vi "app - Ross Thing.vi"() -> ()   [LabVIEW 2012]
uses:
  <vilib>/event_ctls.llb/eventvkey.ctl
  freq file -- file select control.ctl
  freq file -- file select folder control.ctl
  cursor winow.ctl
  fit function selector control.ctl
  countdown control.ctl
  cursor window action.ctl
  container action.ctl
  cursor action.ctl
  save-read action.ctl
  file -- 9w path.vi
  file -- open-create folder.vi
panel:
  in  "main folder":path=path "\\\\rus-one\\newdata/data/Ultrasound/Experiment/ProbeTest/Birdcage/YBCO_6_opt"
  out "Plot: argan":T1(graph)
  in  "Tab : other":enum32{"indicators", "other"}(tab)=enum."other"
  in  "file 2 (red)":T2={"from file "="2011_mo", "load"=TRUE, "read from file list"=3, "folder kind"=enum."monitor"} {"read from file list" items=["795_mo", "1348_mo", "1644_mo", "2011_mo", "2100_mo"]}
  in  "file 1 (blue)":T2={"from file "="2011_mo", "load"=TRUE, "read from file list"=4, "folder kind"=enum."monitor"} {"read from file list" items=["586_mo", "792_mo", "1644_mo", "1865_mo", "2011_mo", "2730_mo"]}
  out "time (min)":dbl=808.9068825910931
  in  "open (o)":bool
  in  "plot (p)":bool
  in  "plot type":T4(ring)=enum."plot vs Temperature"
  out "temperature (K)":dbl=39.718
  out "Magnetic Field (T)":dbl=0.65596
  in  "sweep folder 2":u16(ring)=18 items=["1_test", "2_heating_0T", "3_field_to_5T", "4_cooling_5T", "5_heating_5T", "6_cooling_10T", "7_heating_10T", "8_cooling_1T", "9_heating_2T", "10_test", "11_heating_0T", "12_heating_0T", "14_field_to_5T", "15_field_to_0T", "16_field_to_10T", "17_field_to_0T", "18_field_to_10T", "19_cooling_10T", "20_heating_10T"]
  in  "sweep folder 1":u16(ring)=17 items=["1_test", "2_heating_0T", "3_field_to_5T", "4_cooling_5T", "5_heating_5T", "6_cooling_10T", "7_heating_10T", "8_cooling_1T", "9_heating_2T", "10_test", "11_heating_0T", "12_heating_0T", "14_field_to_5T", "15_field_to_0T", "16_field_to_10T", "17_field_to_0T", "18_field_to_10T", "19_cooling_10T", "20_heating_10T"]
  out "folder --OK":bool=TRUE
  out "file 2 -- OK":bool=TRUE
  out "file 1 -- OK":bool=TRUE
  out "best fit parameters":dbl[](array[numeric])=[2010.73341095214, -73.95493561675569, 194.69833504908257]
  in  "fit dataset":enum16{"fit blue dataset", "fit red  dataset"}(ring)
  in  "fit using":T5=enum."einstein"
  out "current index":dbl=2087.4915004944774
  out "Char":i16=51
  out "VKey":T6
  in  "Tab: timer":enum32{"timer ON", "timer OFF"}(tab)
  in  "timer  \"update\"":dbl(slide)=31059.326000000176 min=-209828747.99999982 max=2129711151.0 step=0.010000000000000002 scale=0.0..300.0 scale format="%#3_3f"
  in  "Tab : all":enum32{"everything", "everything else"}(tab)
  out "Plot: temp vs time":cluster{dbl[], dbl[]}[](graph)
  out "Plot: gamma":cluster{dbl[], dbl[]}[](graph)=[{array[2829 elements], array[2829 elements]}, {[15.988, 15.895, 15.895, 15.863, 15.823, 15.791, 15.753, 15.714, 15.682, 15.645, 15.614, 15.576, 15.545, 15.508, 15.472, 15.441, 15.405, 15.375, 15.339, 15.309, 15.274, 15.245, 15.209, 15.175, 15.146, 15.112, 15.084, 15.05, 15.022, 14.988, 14.96, 14.926, 14.892, 14.864, 14.83, 14.802, 14.769, 14.741, 14.708, 14.675, 14.648, 14.616, 14.589, 14.557, 14.53, 14.499, 14.472, 14.441, 14.41, 14.384, 14.353, 14.327, 14.297, 14.272, 14.242, 14.212, 14.188, 14.158, 14.134, 14.108, 14.091, 14.082, 14.085, 14.104, 14.141, 14.186, 14.259, 14.332, 14.435, 14.532, 14.66, 14.776, 14.923, 15.078, 15.212, 15.375, 15.514, 15.68, 15.818, 15.983, 16.144, 16.275, 16.429, 16.554, 16.697, 16.814, 16.947, 17.054, 17.177, 17.295, 17.39, 17.498, 17.585, 17.685, 17.767, 17.86, 17.951, 18.024, 18.111, 18.181, 18.265, 18.333, 18.415, 18.496, 18.562, 18.643, 18.711, 18.792, 18.861, 18.945, 19.016, 19.102, 19.188, 19.262, 19.352, 19.428, 19.52, 19.598, 19.694, 19.773, 19.87, 19.968, 20.051, 20.151, 20.234, 20.335, 20.419, 20.521, 20.622, 20.706, 20.807, 20.891, 20.992, 21.075, 21.175, 21.258, 21.355, 21.453, 21.534, 21.63, 21.709, 21.804, 21.882, 21.975, 22.068, 22.144, 22.235, 22.31, 22.399, 22.473, 22.562, 22.635, 22.722, 22.81, 22.882, 22.969, 23.041, 23.127, 23.199, 23.285, 23.372, 23.458, 23.545, 23.631, 23.631, 23.717, 23.791, 23.849, 23.922, 23.995, 24.083, 24.157, 24.231, 24.32, 24.394, 24.47, 24.56, 24.635, 24.71, 24.817, 24.924, 25.016, 25.123, 25.216, 25.324, 25.417, 25.526, 25.619, 25.728, 25.821, 25.931, 26.025, 26.134, 26.229, 26.339, 26.448, 26.543, 26.652, 26.746, 26.856, 26.95, 27.06, 27.154, 27.264, 27.359, 27.468, 27.563, 27.673, 27.782, 27.877, 27.987, 28.082, 28.193, 28.288, 28.399, 28.493, 28.605, 28.701, 28.812, 28.909, 29.021, 29.118, 29.231, 29.344, 29.442, 29.556, 29.654, 29.768, 29.868, 29.984, 30.082, 30.2, 30.299, 30.417, 30.518, 30.636, 30.738, 30.857, 30.976, 31.08, 31.2, 31.304, 31.425, 31.529, 31.652, 31.757, 31.881, 31.987, 32.111, 32.217, 32.342, 32.45, 32.576, 32.702, 32.811, 32.938, 33.047, 33.176, 33.286, 33.415, 33.526, 33.656, 33.768, 33.9, 34.012, 34.144, 34.276, 34.391, 34.525, 34.639, 34.773, 34.889], [0.02015, 0.02965, 0.02923, 0.02683, 0.02605, 0.02852, 0.02316, 0.0243, 0.02505, 0.02987, 0.02439, 0.02523, 0.02405, 0.02435, 0.02757, 0.02568, 0.02492, 0.02492, 0.02742, 0.02961, 0.03389, 0.02022, 0.02642, 0.03056, 0.02673, 0.03264, 0.0206, 0.02411, 0.02374, 0.02762, 0.02435, 0.02784, 0.02951, 0.0205, 0.02387, 0.02656, 0.02196, 0.02912, 0.02801, 0.02441, 0.0273, 0.02807, 0.02433, 0.02863, 0.02677, 0.02849, 0.02892, 0.02528, 0.02579, 0.02902, 0.02854, 0.02679, 0.02086, 0.02834, 0.02825, 0.03102, 0.02966, 0.02864, 0.02638, 0.02732, 0.02698, 0.02975, 0.0277, 0.02987, 0.02672, 0.02935, 0.02685, 0.02704, 0.03128, 0.02306, 0.02001, 0.0269, 0.02455, 0.03277, 0.02896, 0.03053, 0.02583, 0.02668, 0.02805, 0.02642, 0.02325, 0.03759, 0.03048, 0.03819, 0.02667, 0.02874, 0.0294, 0.02773, 0.02917, 0.02492, 0.02754, 0.02348, 0.02597, 0.01897, 0.02318, 0.03016, 0.00123, 0.02855, 0.02386, 0.02476, 0.02543, 0.02862, 0.02883, 0.02667, 0.02727, 0.02846, 0.02979, 0.02773, 0.02675, 0.0282, 0.02506, 0.02126, 0.02901, 0.0228, 0.02825, 0.02834, 0.02612, 0.02559, 0.02108, 0.02742, 0.02585, 0.03164, 0.02195, 0.02756, 0.02835, 0.02988, 0.0272, 0.02663, 0.01825, 0.02181, 0.02802, 0.02825, 0.02726, 0.02242, 0.02544, 0.02547, 0.02545, 0.02683, 0.02214, 0.02583, 0.02758, 0.02628, 0.03141, 0.03234, 0.02479, 0.03261, 0.02449, 0.03183, 0.02764, 0.02827, 0.02715, 0.02372, 0.02469, 0.02966, 0.02697, 0.02742, 0.03078, 0.02539, 0.02565, 0.03029, 0.0221, 0.02024, 0.02769, 0.02882, 0.02943, 0.02649, 0.02713, 0.02892, 0.0248, 0.02651, 0.02454, 0.02248, 0.02563, 0.02862, 0.02788, 0.03423, 0.02351, 0.02644, 0.02672, 0.02602, 0.03194, 0.02539, 0.02141, 0.02587, 0.03321, 0.02646, 0.02893, 0.0267, 0.02558, 0.02828, 0.03125, 0.02901, 0.027, 0.02611, 0.03, 0.02445, 0.02946, 0.03169, 0.03087, 0.0278, 0.03122, 0.02918, 0.03277, 0.02628, 0.03193, 0.02932, 0.02643, 0.0297, 0.03219, 0.02259, 0.03189, 0.02575, 0.02956, 0.02823, 0.03083, 0.02432, 0.03081, 0.02805, 0.02895, 0.02949, 0.03329, 0.0252, 0.03217, 0.02851, 0.03302, 0.03135, 0.02939, 0.03259, 0.02891, 0.02694, 0.02764, 0.02818, 0.02816, 0.03219, 0.02872, 0.03218, 0.02862, 0.02924, 0.02826, 0.03453, 0.0286, 0.02929, 0.02829, 0.03049, 0.0285, 0.02886, 0.02983, 0.02924, 0.03279, 0.0299, 0.0307, 0.02869, 0.02945, 0.03194, 0.03101, 0.03509, 0.03178, 0.0325, 0.0284, 0.03111, 0.03673, 0.03112, 0.03366, 0.0325, 0.03392, 0.03124, 0.03357, 0.03122, 0.02909, 0.03521, 0.03121, 0.03304]}]
  out "Plot: field vs time":cluster{dbl[], dbl[]}[](graph)
  out "Plot: frequency":cluster{dbl[], dbl[]}[](graph)=[{array[2829 elements], array[2829 elements]}, {[15.988, 15.895, 15.895, 15.863, 15.823, 15.791, 15.753, 15.714, 15.682, 15.645, 15.614, 15.576, 15.545, 15.508, 15.472, 15.441, 15.405, 15.375, 15.339, 15.309, 15.274, 15.245, 15.209, 15.175, 15.146, 15.112, 15.084, 15.05, 15.022, 14.988, 14.96, 14.926, 14.892, 14.864, 14.83, 14.802, 14.769, 14.741, 14.708, 14.675, 14.648, 14.616, 14.589, 14.557, 14.53, 14.499, 14.472, 14.441, 14.41, 14.384, 14.353, 14.327, 14.297, 14.272, 14.242, 14.212, 14.188, 14.158, 14.134, 14.108, 14.091, 14.082, 14.085, 14.104, 14.141, 14.186, 14.259, 14.332, 14.435, 14.532, 14.66, 14.776, 14.923, 15.078, 15.212, 15.375, 15.514, 15.68, 15.818, 15.983, 16.144, 16.275, 16.429, 16.554, 16.697, 16.814, 16.947, 17.054, 17.177, 17.295, 17.39, 17.498, 17.585, 17.685, 17.767, 17.86, 17.951, 18.024, 18.111, 18.181, 18.265, 18.333, 18.415, 18.496, 18.562, 18.643, 18.711, 18.792, 18.861, 18.945, 19.016, 19.102, 19.188, 19.262, 19.352, 19.428, 19.52, 19.598, 19.694, 19.773, 19.87, 19.968, 20.051, 20.151, 20.234, 20.335, 20.419, 20.521, 20.622, 20.706, 20.807, 20.891, 20.992, 21.075, 21.175, 21.258, 21.355, 21.453, 21.534, 21.63, 21.709, 21.804, 21.882, 21.975, 22.068, 22.144, 22.235, 22.31, 22.399, 22.473, 22.562, 22.635, 22.722, 22.81, 22.882, 22.969, 23.041, 23.127, 23.199, 23.285, 23.372, 23.458, 23.545, 23.631, 23.631, 23.717, 23.791, 23.849, 23.922, 23.995, 24.083, 24.157, 24.231, 24.32, 24.394, 24.47, 24.56, 24.635, 24.71, 24.817, 24.924, 25.016, 25.123, 25.216, 25.324, 25.417, 25.526, 25.619, 25.728, 25.821, 25.931, 26.025, 26.134, 26.229, 26.339, 26.448, 26.543, 26.652, 26.746, 26.856, 26.95, 27.06, 27.154, 27.264, 27.359, 27.468, 27.563, 27.673, 27.782, 27.877, 27.987, 28.082, 28.193, 28.288, 28.399, 28.493, 28.605, 28.701, 28.812, 28.909, 29.021, 29.118, 29.231, 29.344, 29.442, 29.556, 29.654, 29.768, 29.868, 29.984, 30.082, 30.2, 30.299, 30.417, 30.518, 30.636, 30.738, 30.857, 30.976, 31.08, 31.2, 31.304, 31.425, 31.529, 31.652, 31.757, 31.881, 31.987, 32.111, 32.217, 32.342, 32.45, 32.576, 32.702, 32.811, 32.938, 33.047, 33.176, 33.286, 33.415, 33.526, 33.656, 33.768, 33.9, 34.012, 34.144, 34.276, 34.391, 34.525, 34.639, 34.773, 34.889], array[272 elements]}, {array[2829 elements], array[2829 elements]}]
  out "Plot: delta frequency":T7(graph)=[{"Temperature (K) Array"=array[2829 elements], "freq out"=array[2829 elements]}, {"Temperature (K) Array"=[15.988, 15.895, 15.895, 15.863, 15.823, 15.791, 15.753, 15.714, 15.682, 15.645, 15.614, 15.576, 15.545, 15.508, 15.472, 15.441, 15.405, 15.375, 15.339, 15.309, 15.274, 15.245, 15.209, 15.175, 15.146, 15.112, 15.084, 15.05, 15.022, 14.988, 14.96, 14.926, 14.892, 14.864, 14.83, 14.802, 14.769, 14.741, 14.708, 14.675, 14.648, 14.616, 14.589, 14.557, 14.53, 14.499, 14.472, 14.441, 14.41, 14.384, 14.353, 14.327, 14.297, 14.272, 14.242, 14.212, 14.188, 14.158, 14.134, 14.108, 14.091, 14.082, 14.085, 14.104, 14.141, 14.186, 14.259, 14.332, 14.435, 14.532, 14.66, 14.776, 14.923, 15.078, 15.212, 15.375, 15.514, 15.68, 15.818, 15.983, 16.144, 16.275, 16.429, 16.554, 16.697, 16.814, 16.947, 17.054, 17.177, 17.295, 17.39, 17.498, 17.585, 17.685, 17.767, 17.86, 17.951, 18.024, 18.111, 18.181, 18.265, 18.333, 18.415, 18.496, 18.562, 18.643, 18.711, 18.792, 18.861, 18.945, 19.016, 19.102, 19.188, 19.262, 19.352, 19.428, 19.52, 19.598, 19.694, 19.773, 19.87, 19.968, 20.051, 20.151, 20.234, 20.335, 20.419, 20.521, 20.622, 20.706, 20.807, 20.891, 20.992, 21.075, 21.175, 21.258, 21.355, 21.453, 21.534, 21.63, 21.709, 21.804, 21.882, 21.975, 22.068, 22.144, 22.235, 22.31, 22.399, 22.473, 22.562, 22.635, 22.722, 22.81, 22.882, 22.969, 23.041, 23.127, 23.199, 23.285, 23.372, 23.458, 23.545, 23.631, 23.631, 23.717, 23.791, 23.849, 23.922, 23.995, 24.083, 24.157, 24.231, 24.32, 24.394, 24.47, 24.56, 24.635, 24.71, 24.817, 24.924, 25.016, 25.123, 25.216, 25.324, 25.417, 25.526, 25.619, 25.728, 25.821, 25.931, 26.025, 26.134, 26.229, 26.339, 26.448, 26.543, 26.652, 26.746, 26.856, 26.95, 27.06, 27.154, 27.264, 27.359, 27.468, 27.563, 27.673, 27.782, 27.877, 27.987, 28.082, 28.193, 28.288, 28.399, 28.493, 28.605, 28.701, 28.812, 28.909, 29.021, 29.118, 29.231, 29.344, 29.442, 29.556, 29.654, 29.768, 29.868, 29.984, 30.082, 30.2, 30.299, 30.417, 30.518, 30.636, 30.738, 30.857, 30.976, 31.08, 31.2, 31.304, 31.425, 31.529, 31.652, 31.757, 31.881, 31.987, 32.111, 32.217, 32.342, 32.45, 32.576, 32.702, 32.811, 32.938, 33.047, 33.176, 33.286, 33.415, 33.526, 33.656, 33.768, 33.9, 34.012, 34.144, 34.276, 34.391, 34.525, 34.639, 34.773, 34.889], "freq out"=array[272 elements]}]
  in  "file 2 path":path=path "\\\\rus-one\\newdata/data/Ultrasound/Experiment/ProbeTest/Birdcage/YBCO_6_opt/20_heating_10T/9w/monitor/2011_mo.dat"
  in  "file 1 path":path=path "\\\\rus-one\\newdata/data/Ultrasound/Experiment/ProbeTest/Birdcage/YBCO_6_opt/19_cooling_10T/9w/monitor/2011_mo.dat"
  in  "folder 2":path=path "\\\\rus-one\\newdata/data/Ultrasound/Experiment/ProbeTest/Birdcage/YBCO_6_opt/20_heating_10T"
  in  "folder 1":path=path "\\\\rus-one\\newdata/data/Ultrasound/Experiment/ProbeTest/Birdcage/YBCO_6_opt/19_cooling_10T"
  in  "cursor bracket: freq":T8={"left"=20.906, "right "=32.199, "center"=26.5525, "window"=11.293, "cursors"=[1, 2, 3], "relative"=0, "absolute"=0, "fixed vertical offset"=0.0, "vertical offset"=0.0, "skew"=0.0, "default window frac"=0.1, "kind"=enum."symmetric", "skew.left"=0.5, "skew.right"=0.5, "Plot ref"=refnum, "wing order"=enum."forw"}
  in  "cursor bracket: temp vs time":T8={"left"=382.7183695771876, "right "=860.9798618275884, "center"=621.849115702388, "window"=478.2614922504007, "cursors"=[1, 2, 3], "relative"=1, "absolute"=2, "fixed vertical offset"=0.0, "vertical offset"=0.0, "skew"=0.0, "default window frac"=0.1, "kind"=enum."symmetric", "skew.left"=0.5, "skew.right"=0.5, "Plot ref"=refnum, "wing order"=enum."forw"}
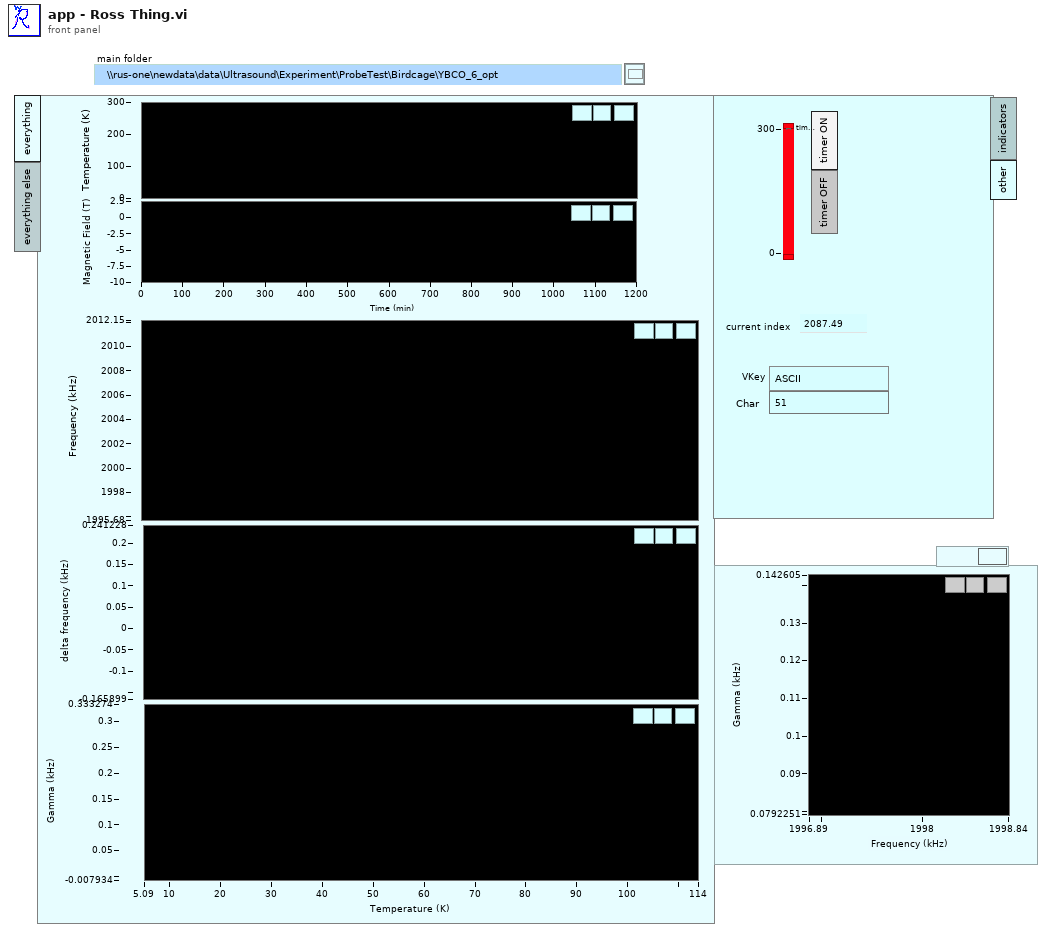
[diagram p1: front panel]
types:
  T1 = cluster{"Frequency (kHz) Array":dbl[], "Gamma (kHz) Array":dbl[]}[]
  T2 = typedef "freq file -- file select control.ctl" = cluster{"from file ":string, "load":bool, "read from file list":u16, "folder kind":T3}
  T3 = typedef "freq file -- file select folder control.ctl" = enum16{"monitor", "9w"}
  T4 = enum16{"plot vs Magnetic Field", "plot vs Temperature"}
  T5 = typedef "fit function selector control.ctl" = enum16{"linear", "varshni", "varshni5", "LogMinusT", "hyperbola", "einstein", "sine", "sine2theta", "cos2theta"}
  T6 = typedef "eventvkey.ctl" = enum16{"ASCII", "Enter", "Return", "Shift", "Ctrl", "Alt", "Cmd", "Opt", "Caps", "NumLock", "Clear", "Break", "Up", "Down", "Left", "Right", "Insert", "Delete", "Home", "End", "PageUp", "PageDown", "Escape", "Help", "Pause", "ScrollLock", "F1", "F2", "F3", "F4", "F5", "F6", "F7", "F8", "F9", "F10", "F11", "F12", "F13", "F14", "F15", "F16", "F17", "F18", "F19", "F20", "F21", "F22", "F23", "F24", "Play", "VolumeUp", "VolumeDown", "Mute", "Two Byte Char"}
  T7 = cluster{"Temperature (K) Array":dbl[], "freq out":dbl[]}[]
  T8 = typedef "cursor winow.ctl" = cluster{"left":dbl, "right ":dbl, "center":dbl, "window":dbl, "cursors":i32[], "relative":i32, "absolute":i32, "fixed vertical offset":dbl, "vertical offset":dbl, "skew":dbl, "default window frac":dbl, "kind":enum16{"symmetric", "skewed", "fancy"}, "skew.left":dbl, "skew.right":dbl, "Plot ref":refnum<vi>, "wing order":enum16{"forw", "back"}}
  T9 = typedef "cursor window action.ctl" = enum16{"balance", "h. offset change", "cursor moves", "change center", "change window", "init", "check", "reset", "set y to middle", "idle", "-write all Y", "-write left.X", "-write center.X", "-write right.X", "-write all X", "-change center", "-change window", "-change skew", "-read cursor 2", "-read cursor 1", "-read cursor 0", "-read all cursors", "-reset", "-read plot scale", "-set y to middle", "-Q: center.Y is visible", "-Q: window is visible", "-parse center.Y", "-right left from center", "-left move", "-right move", "-set center.Y", "-empty", "-set cursors to default", "-check", "-write center.Y", "-copy cursor 1", "-copy cursor 0", "-copy cursor 2", "move right", "move left", "shrink", "broaden", "skew up", "skew down", "-write plot scale", "zoom X", "change cen&win", "zoom to all data"}
  T10 = typedef "countdown control.ctl" = enum16{"check", "start", "reset cont", "stop", "reset once"}
  T11 = typedef "container action.ctl" = enum16{"get", "read file", "plot", "init", "set"}
  T12 = cluster{"time array":dbl[], "Temperature (K) Array":dbl[]}
  T13 = cluster{"time array":dbl[], "Field (T) Array":dbl[]}
  T14 = cluster{"time array":dbl[], "Temperature (K) Array":dbl[]}[]
  T15 = cluster{"time array":dbl[], "Field (T) Array":dbl[]}[]
  T16 = typedef "cursor action.ctl" = enum16{"range", "read", "write", "check", "zoom out", "smart zoom out"}
  T17 = cluster{"Temperature (K) Array":dbl[], "Gamma (kHz) Array":dbl[]}
  T18 = cluster{"Temperature (K) Array":dbl[], "Frequency (kHz) Array":dbl[]}
  T19 = cluster{"Frequency (kHz) Array":dbl[], "Gamma (kHz) Array":dbl[]}
  T20 = cluster{"Temperature (K) Array":dbl[], "Gamma (kHz) Array":dbl[]}[]
  T21 = cluster{"Temperature (K) Array":dbl[], "freq out":dbl[]}
  T22 = cluster{"Field (T) Array":dbl[], "Gamma (kHz) Array":dbl[]}
  T23 = cluster{"Field (T) Array":dbl[], "Frequency (kHz) Array":dbl[]}
  T24 = cluster{"Field (T) Array":dbl[], "Frequency (kHz) Array":dbl[]}[]
  T25 = cluster{"Field (T) Array":dbl[], "Gamma (kHz) Array":dbl[]}[]
  T26 = typedef "save-read action.ctl" = enum16{"update save list", "update read list", "init", "check", "lookup read number", "lookup write number", "copy read from read ring", "saved file dirty", "saved file clean", "read file OK", "read file not OK", "nearest right", "nearest left", "increment read from", "copy read to save", "init save file", "erase event", "save event", "read event", "set save file", "decrement read from"}
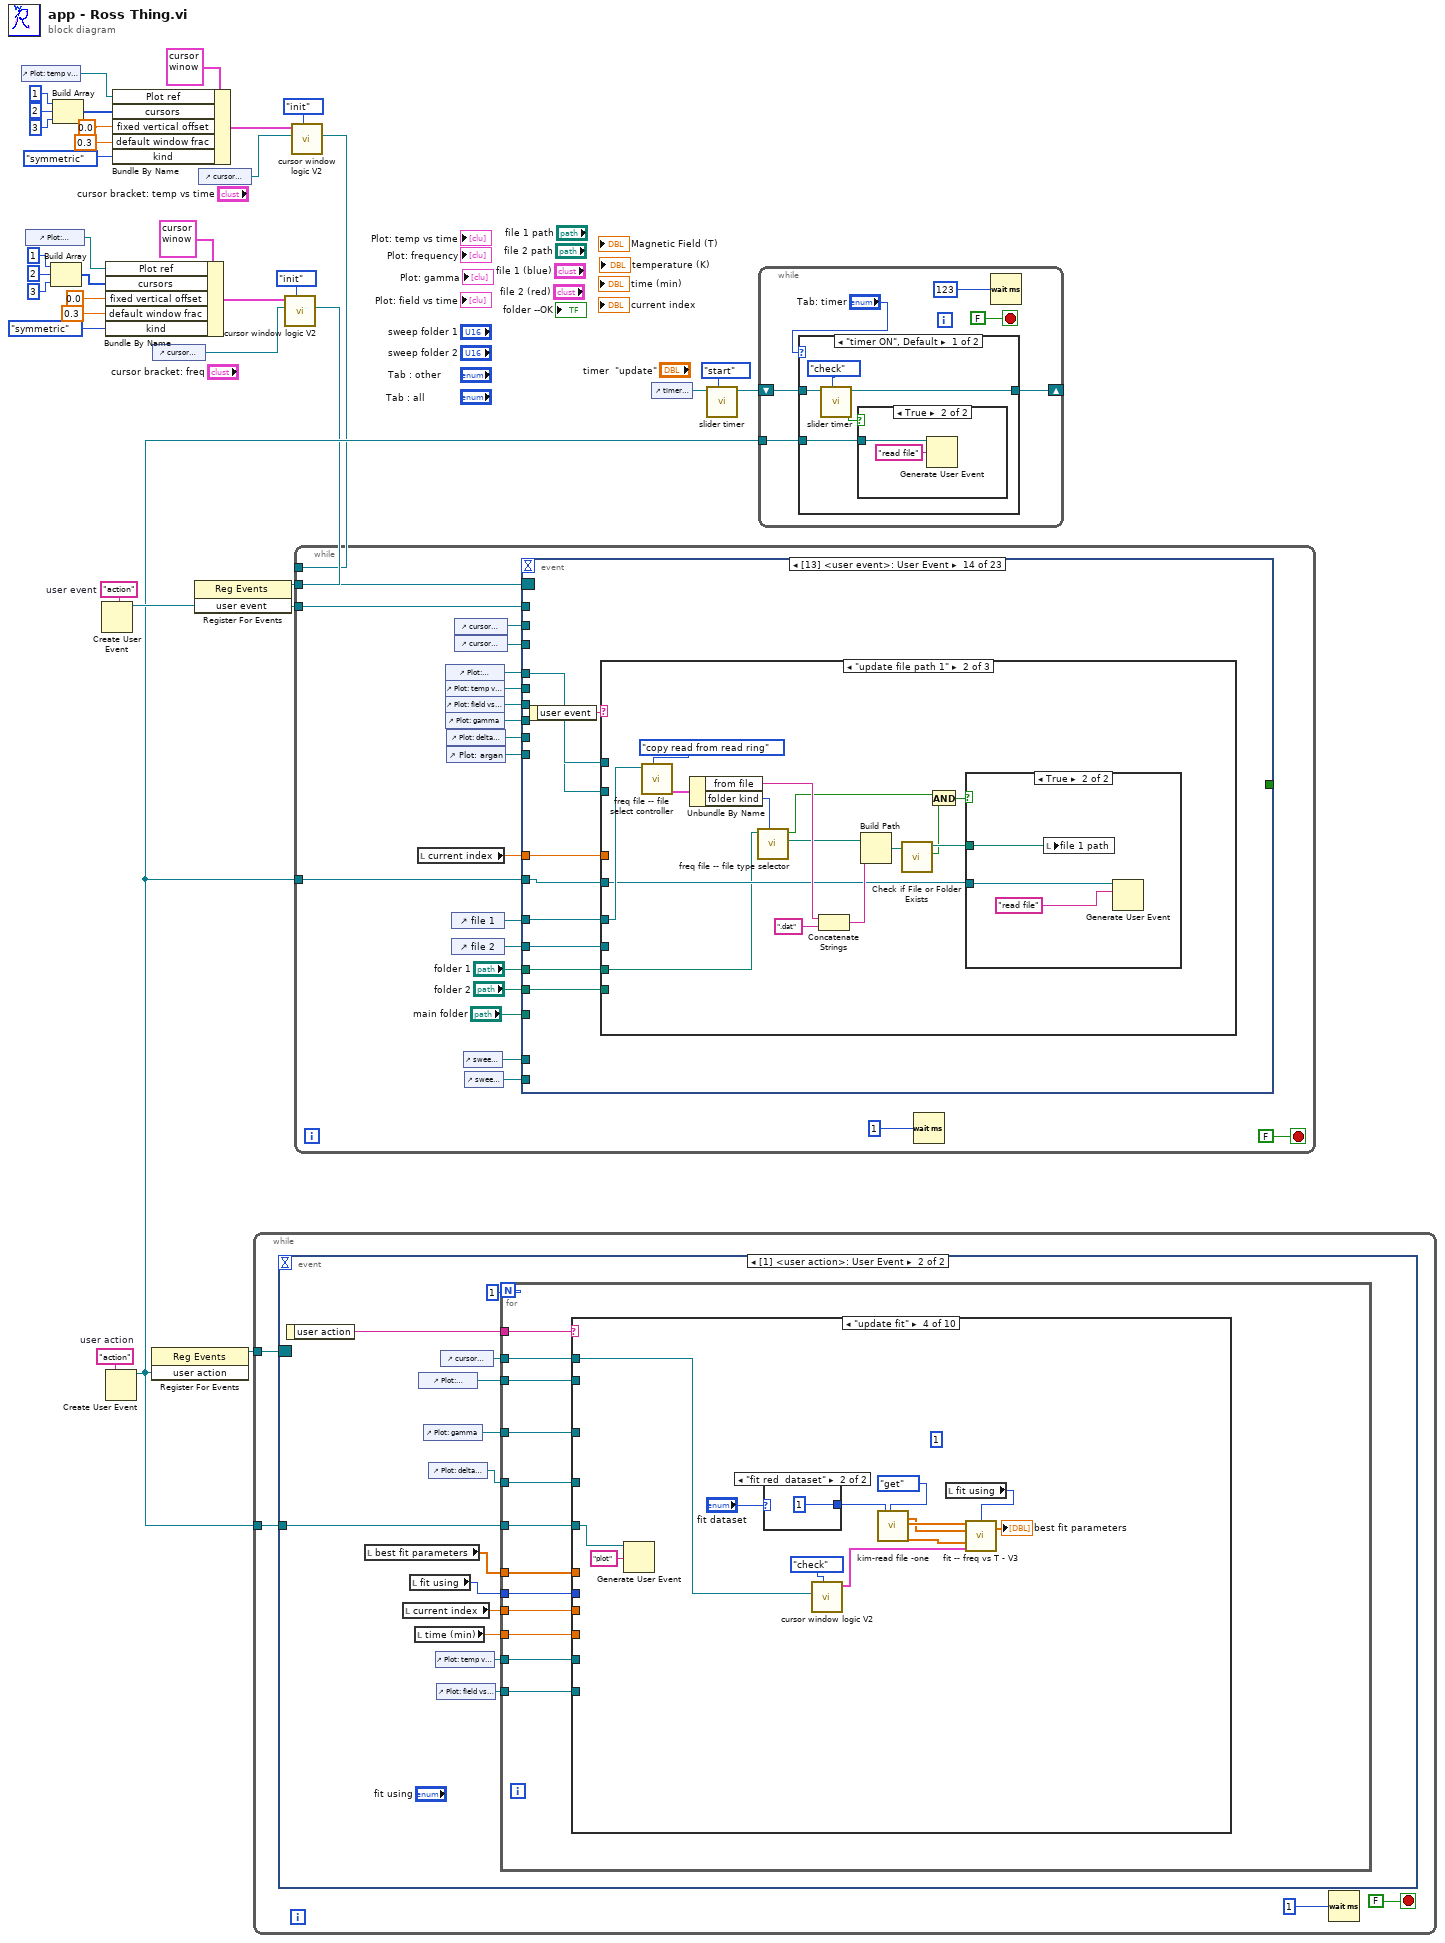
[diagram p0: block diagram]
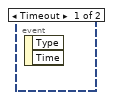
[diagram p4: hidden frame]
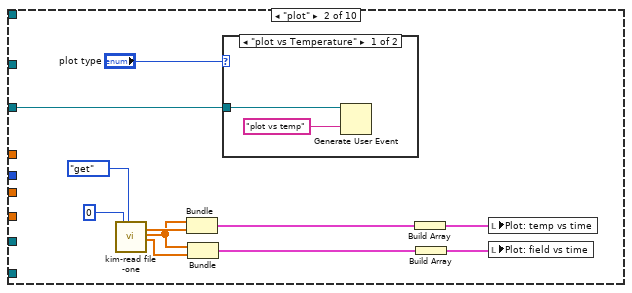
[diagram p6: hidden frame]
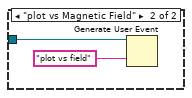
[diagram p7: hidden frame]
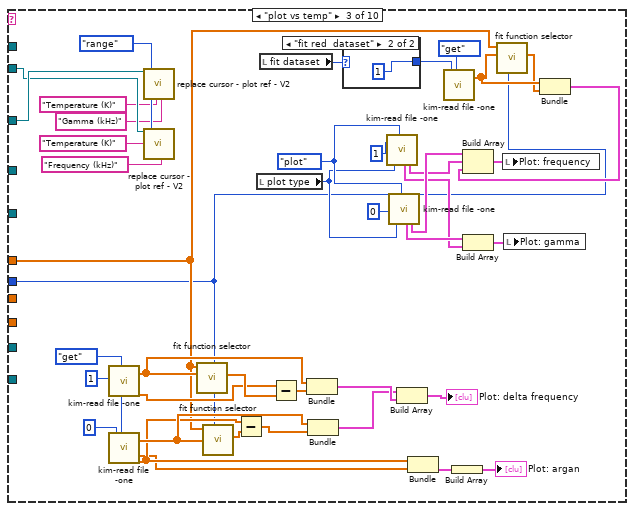
[diagram p8: hidden frame]
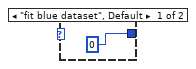
[diagram p9: hidden frame]
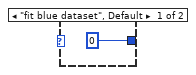
[diagram p10: hidden frame]
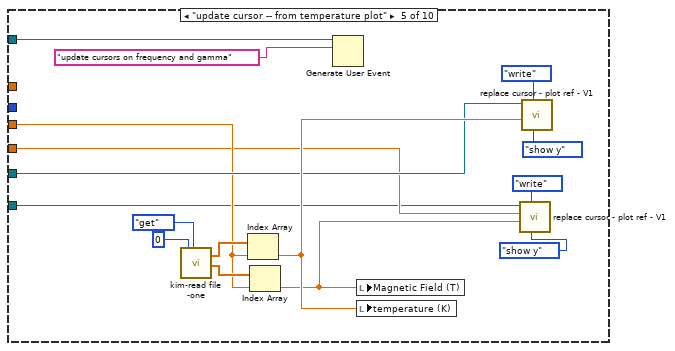
[diagram p11: hidden frame]
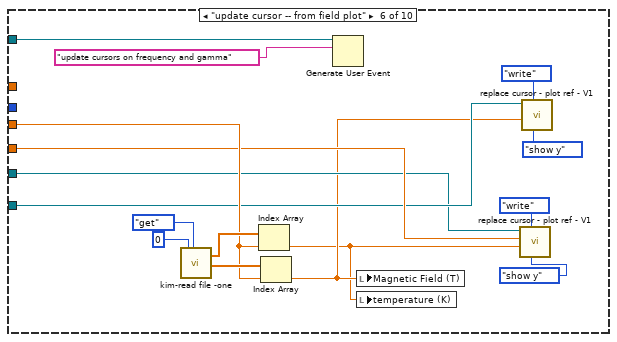
[diagram p12: hidden frame]
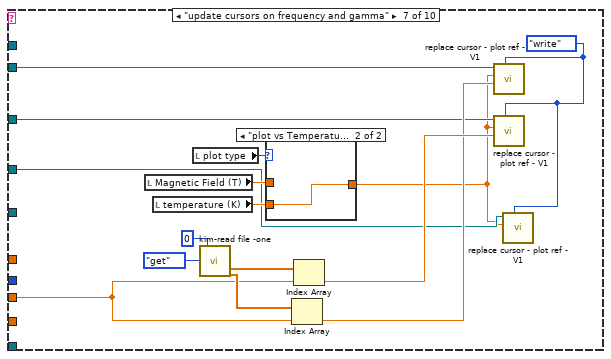
[diagram p13: hidden frame]
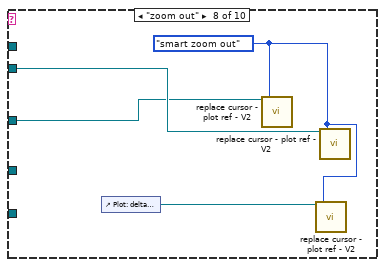
[diagram p15: hidden frame]
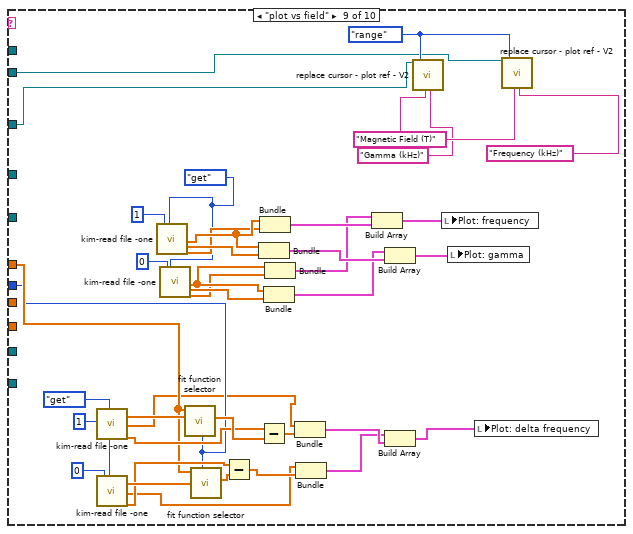
[diagram p16: hidden frame]
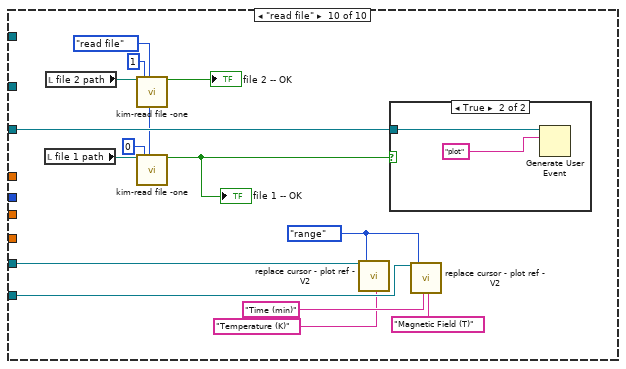
[diagram p17: hidden frame]
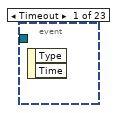
[diagram p19: hidden frame]
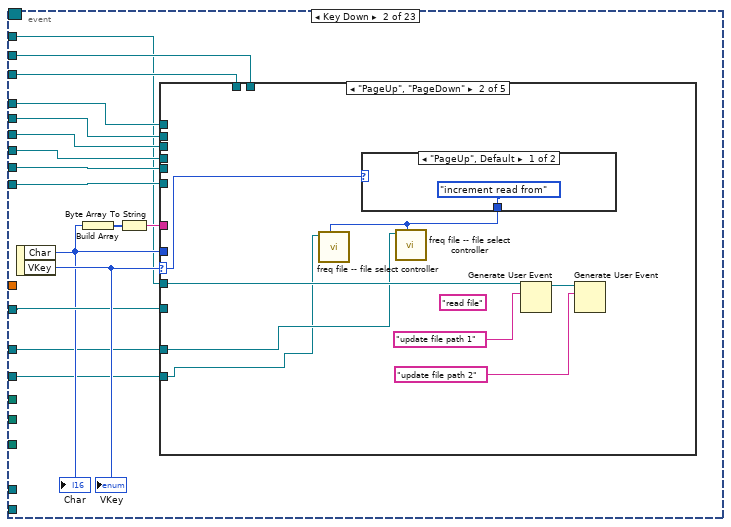
[diagram p20: hidden frame]
diagram:
  w32 = "action"  # user action
  w34 = "action"  # user event
  n1 = control-ref of="Plot: temp vs time"() -> (w6:refnum<vi>)
  n2 = control-ref of="Plot: frequency"() -> (w17:refnum<vi>)
  n3 = Build Array(1, 2, 3) -> (w2:i32[])
  n4 = Build Array(1, 2, 3) -> (w1:i32[])
  n5 = Create User Event(user event datatype=w34) -> (user event=w31:refnum<user-event>)  [unwired: 1 in, 1 out]
  n6 = Bundle By Name(cluster=T8 {"left"=0.0, "right "=0.0, "center"=0.0, "window"=0.0, "cursors"=[], "relative"=0, "absolute"=0, "fixed vertical offset"=0.0, "vertical offset"=0.0, "skew"=0.0, "default window frac"=0.0, "kind"=enum."symmetric", "skew.left"=0.0, "skew.right"=0.0, "Plot ref"=refnum, "wing order"=enum."forw"} ("cursor bracket in"), "Plot ref"=w17, "cursors"=w2, "fixed vertical offset"=0.0, "default window frac"=0.3 ("fixed vertical offset"), "kind"=enum16{"symmetric", "skewed", "fancy"}."symmetric") -> (w26:T8)
  n7 = Create User Event(user event datatype=w32) -> (user event=w28:refnum<user-event>)  [unwired: 1 in, 1 out]
  n8 = Bundle By Name(cluster=T8 {"left"=0.0, "right "=0.0, "center"=0.0, "window"=0.0, "cursors"=[], "relative"=0, "absolute"=0, "fixed vertical offset"=0.0, "vertical offset"=0.0, "skew"=0.0, "default window frac"=0.0, "kind"=enum."symmetric", "skew.left"=0.0, "skew.right"=0.0, "Plot ref"=refnum, "wing order"=enum."forw"} ("cursor bracket in"), "Plot ref"=w6, "cursors"=w1, "fixed vertical offset"=0.0, "default window frac"=0.3 ("fixed vertical offset"), "kind"=enum16{"symmetric", "skewed", "fancy"}."symmetric") -> (w15:T8)
  n9 = register-events(w28) -> (reference out=w33:refnum<event-registration>)  [unwired: 2 in, 1 out]
  n10 = control-ref of="cursor bracket: freq"() -> (w4:refnum<vi>)
  n11 = register-events(w31) -> (reference out=w35:refnum<event-registration>)  [unwired: 2 in, 1 out]
  n12 = control-ref of="cursor bracket: temp vs time"() -> (w3:refnum<vi>)
  n13 = while {
    tunnel: w33 -> [w39]
    tunnel: w28 -> [w36]
    stop <- FALSE stop-if-true
    n14 = event shown="[1] <user action>: User Event" {
      selector: w39 -> [_ _]
      dyn-events: _ -> [_ _]
      timeout: _ -> [_ _]
      tunnel: w36 -> [_ w50]
      event Timeout {
        n15 = event-data() -> ()  [unwired: 1 in, 2 out]
      }
      event User Event {
        n16 = event-data() -> ("user action"=w52:string)  [unwired: 1 in]
        n17 = local read "best fit parameters"() -> (w41:dbl[])
        n18 = local read "current index"() -> (w45:dbl)
        n19 = local read "fit using"() -> (w40:T5)
        n20 = local read "time (min)"() -> (w44:dbl)
        n21 = control-ref of="Plot: frequency"() -> (w48:refnum<vi>)
        n22 = control-ref of="Plot: gamma"() -> (w49:refnum<vi>)
        n23 = control-ref of="Plot: delta frequency"() -> (w43:refnum<vi>)
        n24 = control-ref of="Plot: temp vs time"() -> (w47:refnum<vi>)
        n25 = control-ref of="Plot: field vs time"() -> (w46:refnum<vi>)
        n26 = control-ref of="cursor bracket: temp vs time"() -> (w42:refnum<vi>)
        n27 = for {
          N: 1 -> [_]
          tunnel: w52 -> [w64]
          tunnel: w50 -> [w63]
          tunnel: w49 -> [w62]
          tunnel: w48 -> [w61]
          tunnel: w47 -> [w60]
          tunnel: w46 -> [w59]
          tunnel: w45 -> [w58]
          tunnel: w44 -> [w57]
          tunnel: w43 -> [w56]
          tunnel: w42 -> [w55]
          tunnel: w41 -> [w54]
          tunnel: w40 -> [w53]
          n28 = case shown="\"update fit\"" w64 {
            tunnel: w63 -> [_ w74 _ w125 w141 w160 _ _ _ w244]
            tunnel: w62 -> [_ _ w117 _ _ _ w175 w190 w216 _]
            tunnel: w61 -> [_ _ w114 _ _ _ w176 w191 w213 _]
            tunnel: w60 -> [_ _ _ _ w144 w157 _ _ _ w236]
            tunnel: w59 -> [_ _ _ _ w139 w158 _ _ _ w235]
            tunnel: w58 -> [_ _ _ _ w143 w162 w174 _ _ _]
            tunnel: w57 -> [_ _ _ _ w140 w159 _ _ _ _]
            tunnel: w56 -> [_ _ _ _ _ _ w173 _ _ _]
            tunnel: w55 -> [_ _ _ w124 _ _ _ _ _ _]
            tunnel: w54 -> [_ _ w81 _ _ _ _ _ w196 _]
            tunnel: w53 -> [_ _ w80 _ _ _ _ _ w195 _]
            frame "False", Default {
            }
            frame "plot" {
              n29 = call "kim-read file -one.vi"("Numeric Control"=0, "container action"=container_action."get") -> ("Temperature (K) Array"=w69:dbl[], "time array"=w68:dbl[], "Field (T) Array"=w67:dbl[])  [unwired: 10 in, 5 out]
              n30 = Bundle("time array"=w68, "Temperature (K) Array"=w69) -> (w71:T12)  [unwired: 1 in]
              n31 = Bundle("time array"=w68, "Field (T) Array"=w67) -> (w73:T13)  [unwired: 1 in]
              n32 = case shown="\"plot vs Temperature\"" "plot type" {
                tunnel: w74 -> [w76 w78]
                frame "plot vs Temperature" {
                  n33 = Generate User Event(user event=w76, event data cluster="plot vs temp" ("event data")) -> ()  [unwired: 1 in, 2 out]
                }
                frame "plot vs Magnetic Field" {
                  n34 = Generate User Event(user event=w78, event data cluster="plot vs field" ("event data")) -> ()  [unwired: 1 in, 2 out]
                }
              }
              n35 = Build Array(w71) -> (w70:T14)
              n36 = Build Array(w73) -> (w72:T15)
              n37 = local write "Plot: temp vs time"(w70) -> ()
              n38 = local write "Plot: field vs time"(w72) -> ()
            }
            frame "plot vs temp" {
              w96 = container_action."get" ("container action")
              w113 = cursor_action."range" ("cursor action")
              w118 = container_action."plot" ("container action")
              n39 = call "kim-read file -one.vi"("Numeric Control"=1, "container action"=w96) -> ("Temperature (K) Array"=w98:dbl[], "Frequency (kHz) Array"=w99:dbl[])  [unwired: 10 in, 6 out]
              n40 = call "kim-read file -one.vi"("Numeric Control"=0, "container action"=w96) -> ("Temperature (K) Array"=w95:dbl[], "Gamma (kHz) Array"=w91:dbl[], "Frequency (kHz) Array"=w92:dbl[])  [unwired: 10 in, 5 out]
              n41 = call "replace cursor - plot ref - V2.vi"("Plot ref in"=w117, "cursor action"=w113, "x-label"="Temperature (K)", "y-label"="Gamma (kHz)") -> ()  [unwired: 13 in, 3 out]
              n42 = call "replace cursor - plot ref - V2.vi"("Plot ref in"=w114, "cursor action"=w113, "x-label"="Temperature (K)", "y-label"="Frequency (kHz)") -> ()  [unwired: 13 in, 3 out]
              n43 = call "fit function selector.vi"("fit using"=w80, "temperature"=w98, "best fit parameters"=w81) -> ("freq out"=w104:dbl[])  [unwired: 6 in, 2 out]
              n44 = call "fit function selector.vi"("fit using"=w80, "temperature"=w95, "best fit parameters"=w81) -> ("freq out"=w102:dbl[])  [unwired: 6 in, 2 out]
              n45 = Subtract(x=w92, y=w102) -> (x-y=w101:dbl[])
              n46 = local read "plot type"() -> (w106:T4)
              n47 = local read "fit dataset"() -> (w85:enum16{"fit blue dataset", "fit red  dataset"})
              n48 = Subtract(x=w99, y=w104) -> (x-y=w103:dbl[])
              n49 = Bundle("Temperature (K) Array"=w98, w103) -> (w83:cluster{"Temperature (K) Array":dbl[], dbl[]})  [unwired: 1 in]
              n50 = Bundle("Temperature (K) Array"=w95, w101) -> (w82:cluster{"Temperature (K) Array":dbl[], dbl[]})  [unwired: 1 in]
              n51 = case shown="\"fit red  dataset\"" w85 {
                tunnel: [0 ("Numeric Control") 1 ("Numeric Control")] -> w84
                frame "fit blue dataset", Default {
                }
                frame "fit red  dataset" {
                }
              }
              n52 = call "kim-read file -one.vi"("Numeric Control"=1, "plot type"=w106, "container action"=w118) -> ("Plot linew"=w107:T17, "Plot freq"=w108:T18)  [unwired: 9 in, 6 out]
              n53 = call "kim-read file -one.vi"("Numeric Control"=0, "plot type"=w106, "container action"=w118) -> ("Plot linew"=w109:T17, "Plot freq"=w110:T18)  [unwired: 9 in, 6 out]
              n54 = Build Array(w82, w83) -> (→"Plot: delta frequency":cluster{"Temperature (K) Array":dbl[], dbl[]}[])
              n55 = Bundle("Frequency (kHz) Array"=w92, "Gamma (kHz) Array"=w91) -> (w93:T19)  [unwired: 1 in]
              n56 = call "kim-read file -one.vi"("Numeric Control"=w84, "container action"=container_action."get") -> ("Temperature (K) Array"=w88:dbl[])  [unwired: 10 in, 7 out]
              n57 = Build Array(w93) -> (→"Plot: argan":T1)
              n58 = Build Array(w109, w107) -> (w105:T20)
              n59 = call "fit function selector.vi"("fit using"=w80, "temperature"=w88, "best fit parameters"=w81) -> ("freq out"=w87:dbl[])  [unwired: 6 in, 2 out]
              n60 = local write "Plot: gamma"(w105) -> ()
              n61 = Bundle("Temperature (K) Array"=w88, "freq out"=w87) -> (w86:T21)  [unwired: 1 in]
              n62 = Build Array(w110, w108, w86) -> (w121:T7)
              n63 = local write "Plot: frequency"(w121) -> ()
            }
            frame "update fit" {
              (unwired) 1 ("Numeric Control")
              n64 = Generate User Event(user event=w125, event data cluster="plot" ("event data")) -> ()  [unwired: 1 in, 2 out]
              n65 = case shown="\"fit red  dataset\"" "fit dataset" {
                tunnel: [0 ("Numeric Control") 1 ("Numeric Control")] -> w135
                frame "fit blue dataset", Default {
                }
                frame "fit red  dataset" {
                }
              }
              n66 = call "cursor window logic V2.vi"("cursor window action"=cursor_window_action."check", "cursor window in"=w124) -> ("cursor window out"=w128:T8)  [unwired: 8 in, 1 out]
              n67 = call "kim-read file -one.vi"("Numeric Control"=w135, "container action"=container_action."get") -> ("Temperature (K) Array"=w130:dbl[], "time array"=w136:dbl[], "Frequency (kHz) Array"=w131:dbl[])  [unwired: 10 in, 5 out]
              n68 = local read "fit using"() -> (w133:T5)
              n69 = call "fit -- freq vs T - V3.vi"("time points"=w136, "fit using"=w133, "temperature points"=w130, "frequency points"=w131, "cursor bracket: freq"=w128) -> ("best fit parameters"=→"best fit parameters":dbl[])  [unwired: 7 in, 3 out]
            }
            frame "update cursor -- from temperature plot" {
              n70 = call "kim-read file -one.vi"("Numeric Control"=0, "container action"=container_action."get") -> ("Temperature (K) Array"=w149:dbl[], "Field (T) Array"=w148:dbl[])  [unwired: 10 in, 6 out]
              n71 = Index Array(array=w149, index=w143) -> (element=w146:dbl)
              n72 = Index Array(array=w148, index=w143) -> (element=w145:dbl)
              n73 = Generate User Event(user event=w141, event data cluster="update cursors on frequency and gamma" ("event data")) -> ()  [unwired: 1 in, 2 out]
              n74 = local write "Magnetic Field (T)"(w145) -> ()
              n75 = local write "temperature (K)"(w146) -> ()
              n76 = call "replace cursor - plot ref - V1.vi"("label"=enum16{"hide", "show x", "show y", "show (x,y)"}."show y", "action"=enum16{"", "read", "write"}."write", "new  Y"=w145, "new X"=w140, "Plot ref in"=w139) -> ()  [unwired: 4 in, 3 out]
              n77 = call "replace cursor - plot ref - V1.vi"("label"=enum16{"hide", "show x", "show y", "show (x,y)"}."show y", "action"=enum16{"", "read", "write"}."write", "new  Y"=w146, "Plot ref in"=w144) -> ()  [unwired: 5 in, 3 out]
            }
            frame "update cursor -- from field plot" {
              n78 = call "kim-read file -one.vi"("Numeric Control"=0, "container action"=container_action."get") -> ("Temperature (K) Array"=w165:dbl[], "Field (T) Array"=w164:dbl[])  [unwired: 10 in, 6 out]
              n79 = Index Array(array=w165, index=w162) -> (element=w155:dbl)
              n80 = Index Array(array=w164, index=w162) -> (element=w156:dbl)
              n81 = Generate User Event(user event=w160, event data cluster="update cursors on frequency and gamma" ("event data")) -> ()  [unwired: 1 in, 2 out]
              n82 = local write "Magnetic Field (T)"(w156) -> ()
              n83 = local write "temperature (K)"(w155) -> ()
              n84 = call "replace cursor - plot ref - V1.vi"("label"=enum16{"hide", "show x", "show y", "show (x,y)"}."show y", "action"=enum16{"", "read", "write"}."write", "new  Y"=w155, "new X"=w159, "Plot ref in"=w157) -> ()  [unwired: 4 in, 3 out]
              n85 = call "replace cursor - plot ref - V1.vi"("label"=enum16{"hide", "show x", "show y", "show (x,y)"}."show y", "action"=enum16{"", "read", "write"}."write", "new  Y"=w156, "Plot ref in"=w158) -> ()  [unwired: 5 in, 3 out]
            }
            frame "update cursors on frequency and gamma" {
              w172 = enum16{"", "read", "write"}."write" ("action")
              n86 = local read "Magnetic Field (T)"() -> (w179:dbl)
              n87 = local read "temperature (K)"() -> (w178:dbl)
              n88 = local read "plot type"() -> (w177:T4)
              n89 = call "kim-read file -one.vi"("Numeric Control"=0, "container action"=container_action."get") -> ("Gamma (kHz) Array"=w185:dbl[], "Frequency (kHz) Array"=w182:dbl[])  [unwired: 10 in, 6 out]
              n90 = case shown="\"plot vs Temperature\"" w177 {
                tunnel: [w186 w187] -> w171
                tunnel: w178 -> [_ w187]
                tunnel: w179 -> [w186 _]
                frame "plot vs Magnetic Field", Default {
                }
                frame "plot vs Temperature" {
                }
              }
              n91 = Index Array(array=w182, index=w174) -> (element=w183:dbl)
              n92 = Index Array(array=w185, index=w174) -> (element=w184:dbl)
              n93 = call "replace cursor - plot ref - V1.vi"("action"=w172, "new  Y"=w183, "new X"=w171, "Plot ref in"=w176) -> ()  [unwired: 5 in, 3 out]
              n94 = call "replace cursor - plot ref - V1.vi"("action"=w172, "new  Y"=w184, "new X"=w171, "Plot ref in"=w175) -> ()  [unwired: 5 in, 3 out]
              n95 = call "replace cursor - plot ref - V1.vi"("action"=w172, "new X"=w171, "Plot ref in"=w173) -> ()  [unwired: 6 in, 3 out]
            }
            frame "zoom out" {
              w189 = cursor_action."smart zoom out" ("cursor action")
              n96 = control-ref of="Plot: delta frequency"() -> (w188:refnum<vi>)
              n97 = call "replace cursor - plot ref - V2.vi"("Plot ref in"=w190, "cursor action"=w189) -> ()  [unwired: 15 in, 3 out]
              n98 = call "replace cursor - plot ref - V2.vi"("Plot ref in"=w188, "cursor action"=w189) -> ()  [unwired: 15 in, 3 out]
              n99 = call "replace cursor - plot ref - V2.vi"("Plot ref in"=w191, "cursor action"=w189) -> ()  [unwired: 15 in, 3 out]
            }
            frame "plot vs field" {
              w201 = container_action."get" ("container action")
              w217 = cursor_action."range" ("cursor action")
              w218 = container_action."get" ("container action")
              w215 = "Magnetic Field (T)"
              n100 = call "kim-read file -one.vi"("Numeric Control"=1, "container action"=w201) -> ("Temperature (K) Array"=w203:dbl[], "Field (T) Array"=w193:dbl[], "Frequency (kHz) Array"=w204:dbl[])  [unwired: 10 in, 5 out]
              n101 = call "kim-read file -one.vi"("Numeric Control"=0, "container action"=w201) -> ("Temperature (K) Array"=w200:dbl[], "Field (T) Array"=w192:dbl[], "Frequency (kHz) Array"=w199:dbl[])  [unwired: 10 in, 5 out]
              n102 = call "kim-read file -one.vi"("Numeric Control"=1, "container action"=w218) -> ("Field (T) Array"=w224:dbl[], "Gamma (kHz) Array"=w223:dbl[], "Frequency (kHz) Array"=w222:dbl[])  [unwired: 10 in, 5 out]
              n103 = call "kim-read file -one.vi"("Numeric Control"=0, "container action"=w218) -> ("Field (T) Array"=w221:dbl[], "Gamma (kHz) Array"=w220:dbl[], "Frequency (kHz) Array"=w219:dbl[])  [unwired: 10 in, 5 out]
              n104 = call "fit function selector.vi"("fit using"=w195, "temperature"=w203, "best fit parameters"=w196) -> ("freq out"=w209:dbl[])  [unwired: 6 in, 2 out]
              n105 = call "fit function selector.vi"("fit using"=w195, "temperature"=w200, "best fit parameters"=w196) -> ("freq out"=w207:dbl[])  [unwired: 6 in, 2 out]
              n106 = Subtract(x=w199, y=w207) -> (x-y=w206:dbl[])
              n107 = Bundle("Field (T) Array"=w224, "Gamma (kHz) Array"=w223) -> (w229:T22)  [unwired: 1 in]
              n108 = Subtract(x=w204, y=w209) -> (x-y=w208:dbl[])
              n109 = Bundle("Field (T) Array"=w224, "Frequency (kHz) Array"=w222) -> (w230:T23)  [unwired: 1 in]
              n110 = Bundle("Field (T) Array"=w221, "Gamma (kHz) Array"=w220) -> (w210:T22)  [unwired: 1 in]
              n111 = Bundle("Field (T) Array"=w221, "Frequency (kHz) Array"=w219) -> (w211:T23)  [unwired: 1 in]
              n112 = Bundle("Field (T) Array"=w193, w208) -> (w198:cluster{"Field (T) Array":dbl[], dbl[]})  [unwired: 1 in]
              n113 = Bundle("Field (T) Array"=w192, w206) -> (w197:cluster{"Field (T) Array":dbl[], dbl[]})  [unwired: 1 in]
              n114 = Build Array(w211, w230) -> (w227:T24)
              n115 = Build Array(w210, w229) -> (w228:T25)
              n116 = Build Array(w197, w198) -> (w194:cluster{"Field (T) Array":dbl[], dbl[]}[])
              n117 = call "replace cursor - plot ref - V2.vi"("Plot ref in"=w216, "cursor action"=w217, "x-label"=w215, "y-label"="Gamma (kHz)") -> ()  [unwired: 13 in, 3 out]
              n118 = local write "Plot: frequency"(w227) -> ()
              n119 = local write "Plot: gamma"(w228) -> ()
              n120 = local write "Plot: delta frequency"(w194) -> ()
              n121 = call "replace cursor - plot ref - V2.vi"("Plot ref in"=w213, "cursor action"=w217, "x-label"=w215, "y-label"="Frequency (kHz)") -> ()  [unwired: 13 in, 3 out]
            }
            frame "read file" {
              w239 = container_action."read file" ("container action")
              w234 = cursor_action."range" ("cursor action")
              n122 = local read "file 1 path"() -> (w237:path)
              n123 = local read "file 2 path"() -> (w238:path)
              n124 = call "kim-read file -one.vi"("File Path Control"=w238, "Numeric Control"=1, "container action"=w239) -> ("OK?"=→"file 2 -- OK":bool)  [unwired: 9 in, 7 out]
              n125 = call "kim-read file -one.vi"("File Path Control"=w237, "Numeric Control"=0, "container action"=w239) -> ("OK?"=w242:bool)  [unwired: 9 in, 7 out]
              "file 1 -- OK" <- w242
              n126 = call "replace cursor - plot ref - V2.vi"("Plot ref in"=w236, "cursor action"=w234, "y-label"="Temperature (K)" ("x-label")) -> ()  [unwired: 14 in, 3 out]
              n127 = case shown="True" w242 {
                tunnel: w244 -> [_ w245]
                frame False {
                }
                frame True {
                  n128 = Generate User Event(user event=w245, event data cluster="plot" ("event data")) -> ()  [unwired: 1 in, 2 out]
                }
              }
              n129 = call "replace cursor - plot ref - V2.vi"("Plot ref in"=w235, "cursor action"=w234, "x-label"="Time (min)", "y-label"="Magnetic Field (T)" ("x-label")) -> ()  [unwired: 13 in, 3 out]
            }
          }
        }
      }
    }
    n130 = Wait (ms)(milliseconds to wait=u32 1) -> ()  [unwired: 1 out]
  }
  n131 = call "cursor window logic V2.vi"("cursor window action"=cursor_window_action."init", "cursor window in"=w4, "cursor window init"=w26) -> ("cursor window out"=w16:refnum<vi>)  [unwired: 7 in, 1 out]
  n132 = call "cursor window logic V2.vi"("cursor window action"=cursor_window_action."init", "cursor window in"=w3, "cursor window init"=w15) -> ("cursor window out"=w5:refnum<vi>)  [unwired: 7 in, 1 out]
  n133 = while {
    tunnel: w35 -> [w267]
    tunnel: w28 -> [w264]
    tunnel: w31 -> [w260]
    tunnel: w16 -> [_]
    tunnel: w5 -> [_]
    stop <- FALSE stop-if-true
    n134 = local read "current index"() -> (w258:dbl)
    n135 = control-ref of="Plot: frequency"() -> (w262:refnum<vi>)
    n136 = control-ref of="Plot: temp vs time"() -> (w259:refnum<vi>)
    n137 = control-ref of="Plot: field vs time"() -> (w263:refnum<vi>)
    n138 = control-ref of="Plot: gamma"() -> (w261:refnum<vi>)
    n139 = control-ref of="Plot: delta frequency"() -> (w249:refnum<vi>)
    n140 = control-ref of="Plot: argan"() -> (w247:refnum<vi>)
    n141 = control-ref of="file 1"() -> (w255:refnum<vi>)
    n142 = control-ref of="file 2"() -> (w254:refnum<vi>)
    n143 = control-ref of="cursor bracket: temp vs time"() -> (w250:refnum<vi>)
    n144 = control-ref of="cursor bracket: freq"() -> (w248:refnum<vi>)
    n145 = control-ref of="sweep folder 1"() -> (w251:refnum<vi>)
    n146 = control-ref of="sweep folder 2"() -> (w252:refnum<vi>)
    n147 = event shown="[13] <user event>: User Event" {
      selector: w267 -> [_ _ _ _ _ _ _ _ _ _ _ _ _ _ _ _ _ _ _ _ _ _ _]
      dyn-events: _ -> [_ _ _ _ _ _ _ _ _ _ _ _ _ _ _ _ _ _ _ _ _ _ _]
      timeout: _ -> [_ _ _ _ _ _ _ _ _ _ _ _ _ _ _ _ _ _ _ _ _ _ _]
      tunnel: [_ _ _ _ _ _ _ _ _ _ _ _ _ _ _ _ _ _ _ _ _ "plot (p)" "open (o)"] -> _
      tunnel: w264 -> [_ w282 _ w345 _ _ _ _ _ w370 w375 w378 w380 w385 _ _ _ w455 _ _ w476 w510 w513]
      tunnel: w263 -> [_ w278 _ _ _ _ _ _ _ _ _ _ _ _ _ _ _ _ _ w472 _ _ _]
      tunnel: w262 -> [_ w277 _ _ _ _ _ _ _ _ _ _ _ w390 _ _ _ _ _ _ _ _ _]
      tunnel: w261 -> [_ w276 _ _ _ _ _ _ _ _ _ _ _ w389 _ _ _ _ _ _ _ _ _]
      tunnel: w260 -> [_ w268 _ _ _ _ _ w366 w368 _ _ _ _ _ _ _ w447 _ w457 w470 _ _ _]
      tunnel: w259 -> [_ w279 _ _ _ _ _ _ _ _ _ _ _ _ _ _ _ _ _ _ w478 _ _]
      tunnel: w258 -> [_ _ _ _ _ _ _ _ _ _ _ _ _ w387 _ _ _ _ _ _ _ _ _]
      tunnel: w255 -> [_ w270 _ _ _ w359 _ _ _ w373 _ _ _ w386 _ _ _ _ _ _ _ _ _]
      tunnel: w254 -> [_ w269 _ _ _ _ w362 _ _ _ w374 _ _ w382 _ _ _ _ _ _ _ _ _]
      tunnel: "folder 1" -> [_ _ _ _ _ w356 _ _ _ _ _ _ _ w384 _ _ _ _ _ _ _ _ _]
      tunnel: "folder 2" -> [_ _ _ _ _ _ w361 _ _ _ _ _ _ w383 _ _ _ _ _ _ _ _ _]
      tunnel: "main folder" -> [_ _ _ _ _ _ _ _ _ _ _ _ _ _ w430 w440 w451 _ w462 _ _ _ _]
      tunnel: w252 -> [_ _ _ _ _ _ _ _ _ _ _ _ _ _ w428 _ _ _ w459 _ _ _ _]
      tunnel: w251 -> [_ _ _ _ _ _ _ _ _ _ _ _ _ _ _ w438 w454 _ _ _ _ _ _]
      tunnel: w248 -> [_ w281 w342 _ _ _ _ _ _ _ _ _ _ _ _ _ _ _ _ _ w474 _ _]
      tunnel: w250 -> [_ w280 _ w347 _ _ _ _ _ _ _ _ _ _ _ _ _ _ _ _ w475 _ _]
      tunnel: w249 -> [_ w275 _ _ _ _ _ _ _ _ _ _ _ _ _ _ _ _ _ _ _ _ _]
      tunnel: w247 -> [_ w271 _ _ _ _ _ _ _ _ _ _ _ _ _ _ _ _ _ _ _ _ _]
      event Timeout {
        n148 = event-data() -> ()  [unwired: 1 in, 2 out]
      }
      event Key Down {
        n149 = event-data() -> ("Char"=w274:i16, "VKey"=w283:T6)  [unwired: 1 in]
        "Char" <- w274
        "VKey" <- w283
        n150 = Build Array(w274) -> (w273:i16[])
        n151 = Byte Array To String(unsigned byte array=w273) -> (string=w272:string)
        n152 = case shown="\"PageUp\", \"PageDown\"" w283 {
          selector: w283 -> [_ w304 _ _ w329]
          tunnel: w274 -> [_ _ _ _ _]
          tunnel: w282 -> [w290 _ _ _ w326]
          tunnel: w281 -> [w289 _ _ _ _]
          tunnel: w280 -> [w288 _ _ _ w328]
          tunnel: w277 -> [_ _ w320 _ _]
          tunnel: w279 -> [_ _ w319 _ _]
          tunnel: w278 -> [_ _ w318 _ _]
          tunnel: w276 -> [_ _ w317 _ _]
          tunnel: w275 -> [_ _ w312 _ _]
          tunnel: w272 -> [w287 _ _ _ _]
          tunnel: w271 -> [_ _ w311 _ _]
          tunnel: w270 -> [w286 w302 _ _ _]
          tunnel: w269 -> [w285 w301 _ _ _]
          tunnel: w268 -> [w284 w303 _ _ _]
          frame "ASCII", Default {
            n153 = case shown="\"z\"" w287 {
              tunnel: w290 -> [_ w291 w293 w295 _ _]
              tunnel: w289 -> [_ _ _ _ _ w298]
              tunnel: w288 -> [_ _ _ _ _ w297]
              tunnel: w286 -> [_ _ _ _ _ _]
              tunnel: w285 -> [_ _ _ _ _ _]
              tunnel: w284 -> [_ _ _ _ _ _]
              frame "0", Default {
              }
              frame "p" {
                # "p"
                n154 = Generate User Event(user event=w291, event data cluster="plot" ("event data")) -> ()  [unwired: 1 in, 2 out]
              }
              frame " ", "o" {
                # "<space>"
                # "o"
                n155 = Generate User Event(user event=w293, event data cluster="read file" ("event data")) -> ()  [unwired: 1 in, 2 out]
              }
              frame "z" {
                # "z"
                n156 = Generate User Event(user event=w295, event data cluster="zoom out" ("event data")) -> ()  [unwired: 1 in, 2 out]
              }
              frame "A", "a" {
              }
              frame "c" {
                # "c"
                n157 = call "cursor window logic V2.vi"("cursor window action"=cursor_window_action."check", "cursor window in"=w297) -> ()  [unwired: 8 in, 2 out]
                n158 = call "cursor window logic V2.vi"("cursor window action"=cursor_window_action."check", "cursor window in"=w298) -> ()  [unwired: 8 in, 2 out]
              }
            }
          }
          frame "PageUp", "PageDown" {
            (unwired) "read file" ("event data")
            n159 = case shown="\"PageUp\", Default" w304 {
              tunnel: [save-read_action."increment read from" ("action") save-read_action."decrement read from" ("action")] -> w308
              frame "PageUp", Default {
              }
              frame "PageDown" {
              }
            }
            n160 = call "freq file -- file select controller.vi"("action"=w308, "file select ref"=w301) -> ()  [unwired: 7 in, 3 out]
            n161 = call "freq file -- file select controller.vi"("action"=w308, "file select ref"=w302) -> ()  [unwired: 7 in, 3 out]
            n162 = Generate User Event(user event=w303, event data cluster="update file path 1" ("event data")) -> (user event out=w306:refnum<user-event>)  [unwired: 1 in, 1 out]
            n163 = Generate User Event(user event=w306, event data cluster="update file path 2" ("event data")) -> ()  [unwired: 1 in, 2 out]
          }
          frame "Escape" {
            n164 = Build Array(w320, w319, w318, w317, w312, w311) -> (w316:refnum<vi>[])
            n165 = for {
              tunnel: w316 -> [w325] mode=indexing
              tunnel: [w324] -> w315
              tunnel: [w323] -> w313 mode=indexing
              n166 = property class="XYGraph (strict)"(reference=w325) -> (reference out=w323:refnum<vi>, "Palette Visible"=w324:bool)  [unwired: 1 in, 1 out]
            }
            n167 = Not(x=w315) -> (.not. x?=w314:bool)
            n168 = for {
              tunnel: w314 -> [w322]
              tunnel: w313 -> [w321] mode=indexing
              n169 = property class="XYGraph (strict)"(reference=w321, "Palette Visible"=w322) -> ()  [unwired: 1 in, 2 out]
            }
          }
          frame "Enter" {
          }
          frame "Up".."Right" {
            n170 = case shown="\"Down\"" w329 {
              tunnel: w328 -> [w330 w332 w334 w336 w338 w341]
              frame "Right", Default {
                n171 = call "cursor window logic V2.vi"("cursor window action"=cursor_window_action."move right", "cursor window in"=w330) -> ()  [unwired: 8 in, 2 out]
              }
              frame "Left" {
                n172 = call "cursor window logic V2.vi"("cursor window action"=cursor_window_action."move left", "cursor window in"=w332) -> ()  [unwired: 8 in, 2 out]
              }
              frame "PageUp" {
                n173 = call "cursor window logic V2.vi"("cursor window action"=cursor_window_action."skew up", "cursor window in"=w334) -> ()  [unwired: 8 in, 2 out]
              }
              frame "PageDown" {
                n174 = call "cursor window logic V2.vi"("cursor window action"=cursor_window_action."skew down", "cursor window in"=w336) -> ()  [unwired: 8 in, 2 out]
              }
              frame "Up" {
                n175 = call "cursor window logic V2.vi"("cursor window action"=cursor_window_action."broaden", "cursor window in"=w338) -> ()  [unwired: 8 in, 2 out]
              }
              frame "Down" {
                n176 = call "cursor window logic V2.vi"("cursor window action"=cursor_window_action."shrink", "cursor window in"=w341) -> ()  [unwired: 8 in, 2 out]
              }
            }
            n177 = Generate User Event(user event=w326, event data cluster="update fit" ("event data")) -> ()  [unwired: 1 in, 2 out]
          }
        }
      }
      event "Plot: frequency": Cursor Move {
        n178 = event-data() -> ("CursIdx"=w343:i32)  [unwired: 1 in, 3 out]
        n179 = call "cursor window logic V2.vi"("CursIdx"=w343, "cursor window action"=cursor_window_action."cursor moves", "cursor window in"=w342) -> ()  [unwired: 7 in, 2 out]
      }
      event "Plot: temp vs time": Cursor Release {
        n180 = event-data() -> ("CursIdx"=w346:i32)  [unwired: 1 in, 3 out]
        n181 = case shown="2..4" w346 {
          tunnel: w347 -> [_ _]
          tunnel: w345 -> [_ w348]
          frame 0, Default {
          }
          frame 2..4 {
            n182 = Generate User Event(user event=w348, event data cluster="update fit" ("event data")) -> ()  [unwired: 1 in, 2 out]
          }
        }
      }
      event "fit dataset": Value Change {
        n183 = event-data() -> ("NewVal"=w353:enum16{"fit blue dataset", "fit red  dataset"})  [unwired: 1 in]
        n184 = case shown="\"fit blue dataset\", Default" w353 {
          tunnel: [u32 11589887 u32 16752849] -> w350
          frame "fit blue dataset", Default {
          }
          frame "fit red  dataset" {
          }
        }
        n185 = control-ref of="fit dataset"() -> (w352:refnum<vi>)
        n186 = property class="Enum (strict)"(reference=w352, "RingText.BGColor"=w350, "RingText.TextColor"=u32 460551) -> ()  [unwired: 1 in, 2 out]
      }
      event Mouse Enter {
        n187 = event-data() -> ()  [unwired: 1 in, 1 out]
        n188 = call "freq file -- file select controller.vi"("Sweep folder path"=w356, "action"=save-read_action."update read list", "file select ref"=w359) -> ("file select ref out"=w357:refnum<vi>)  [unwired: 6 in, 2 out]
        n189 = call "freq file -- file select controller.vi"("action"=save-read_action."copy read from read ring", "file select ref"=w357) -> ()  [unwired: 7 in, 3 out]
      }
      event Mouse Enter {
        n190 = event-data() -> ()  [unwired: 1 in, 4 out]
        n191 = call "freq file -- file select controller.vi"("Sweep folder path"=w361, "action"=save-read_action."update read list", "file select ref"=w362) -> ("file select ref out"=w363:refnum<vi>)  [unwired: 6 in, 2 out]
        n192 = call "freq file -- file select controller.vi"("action"=save-read_action."copy read from read ring", "file select ref"=w363) -> ()  [unwired: 7 in, 3 out]
      }
      event Value Change; Mouse Down {
        n193 = event-data() -> ()  [unwired: 1 in, 1 out]
        n194 = Generate User Event(user event=w366, event data cluster="update file path 1" ("event data")) -> ()  [unwired: 1 in, 2 out]
      }
      event Value Change; Mouse Down {
        n195 = event-data() -> ()  [unwired: 1 in, 2 out]
        n196 = Generate User Event(user event=w368, event data cluster="update file path 2" ("event data")) -> ()  [unwired: 1 in, 2 out]
      }
      event Value Change {
        n197 = event-data() -> ()  [unwired: 1 in, 1 out]
        n198 = call "freq file -- file select controller.vi"("action"=save-read_action."read event", "file select ref"=w373) -> ()  [unwired: 7 in, 3 out]
        n199 = Generate User Event(user event=w370, event data cluster="read file" ("event data")) -> ()  [unwired: 1 in, 2 out]
      }
      event Value Change {
        n200 = event-data() -> ()  [unwired: 1 in, 1 out]
        n201 = call "freq file -- file select controller.vi"("action"=save-read_action."read event", "file select ref"=w374) -> ()  [unwired: 7 in, 3 out]
        n202 = Generate User Event(user event=w375, event data cluster="read file" ("event data")) -> ()  [unwired: 1 in, 2 out]
      }
      event "file 1 path", "file 2 path": Value Change {
        n203 = event-data() -> ()  [unwired: 1 in, 1 out]
        n204 = Generate User Event(user event=w378, event data cluster="read file" ("event data")) -> ()  [unwired: 1 in, 2 out]
      }
      event "plot type": Value Change {
        n205 = event-data() -> ()  [unwired: 1 in, 1 out]
        n206 = Generate User Event(user event=w380, event data cluster="plot" ("event data")) -> ()  [unwired: 1 in, 2 out]
      }
      event User Event {
        n207 = event-data() -> ("user event"=w388:string)  [unwired: 1 in]
        n208 = case shown="\"update file path 1\"" w388 {
          tunnel: w390 -> [_ _ _]
          tunnel: w389 -> [_ _ _]
          tunnel: w387 -> [_ _ _]
          tunnel: w386 -> [_ w396 _]
          tunnel: w385 -> [_ w395 w414]
          tunnel: w384 -> [_ w394 _]
          tunnel: w383 -> [_ _ w413]
          tunnel: w382 -> [_ _ w412]
          frame "False", Default {
          }
          frame "update file path 1" {
            n209 = call "freq file -- file select controller.vi"("action"=save-read_action."copy read from read ring", "file select ref"=w396) -> ("file select OUT"=w404:T2)  [unwired: 7 in, 2 out]
            n210 = Unbundle By Name(w404) -> ("from file"=w400:string, "folder kind"=w399:T3)
            n211 = call "freq file -- file type selector.vi"("folder kind"=w399, "Sweep folder path"=w394) -> ("folder path"=w398:path, "OK"=w392:bool)  [unwired: 7 in, 1 out]
            n212 = Concatenate Strings(w400, ".dat" ("name or relative path")) -> (w403:string)
            n213 = Build Path(base path=w398, name or relative path=w403) -> (appended path=w401:path)
            n214 = call <vilib>:"Check if File or Folder Exists.vi"("path"=w401) -> ("file or folder exists?"=w393:bool, "dup path"=w397:path)  [unwired: 8 in, 1 out]
            n215 = And(x=w392, y=w393) -> (x .and. y?=w391:bool)
            n216 = case shown="True" w391 {
              tunnel: w397 -> [_ w406]
              tunnel: w395 -> [_ w407]
              frame False {
              }
              frame True {
                n217 = local write "file 1 path"(w406) -> ()
                n218 = Generate User Event(user event=w407, event data cluster="read file" ("event data")) -> ()  [unwired: 1 in, 2 out]
              }
            }
          }
          frame "update file path 2" {
            n219 = call "freq file -- file select controller.vi"("action"=save-read_action."copy read from read ring", "file select ref"=w412) -> ("file select OUT"=w422:T2)  [unwired: 7 in, 2 out]
            n220 = Unbundle By Name(w422) -> ("from file"=w418:string, "folder kind"=w417:T3)
            n221 = call "freq file -- file type selector.vi"("folder kind"=w417, "Sweep folder path"=w413) -> ("folder path"=w416:path, "OK"=w410:bool)  [unwired: 7 in, 1 out]
            n222 = Concatenate Strings(w418, ".dat" ("name or relative path")) -> (w421:string)
            n223 = Build Path(base path=w416, name or relative path=w421) -> (appended path=w419:path)
            n224 = call <vilib>:"Check if File or Folder Exists.vi"("path"=w419) -> ("file or folder exists?"=w411:bool, "dup path"=w415:path)  [unwired: 8 in, 1 out]
            n225 = And(x=w410, y=w411) -> (x .and. y?=w409:bool)
            n226 = case shown="True" w409 {
              tunnel: w415 -> [_ w424]
              tunnel: w414 -> [_ w425]
              frame False {
              }
              frame True {
                n227 = local write "file 2 path"(w424) -> ()
                n228 = Generate User Event(user event=w425, event data cluster="read file" ("event data")) -> ()  [unwired: 1 in, 2 out]
              }
            }
          }
        }
      }
      event "sweep folder 2": Mouse Enter {
        n229 = event-data() -> ()  [unwired: 1 in, 1 out]
        n230 = call "list - get folder names.vi"("Numeric sort?"=TRUE, "folder path"=w430) -> ("Array"=w431:string[], "OK"=w432:bool)  [unwired: 8 in]
        n231 = case shown="False" w432 {
          selector: w432 -> [w433 w434]
          tunnel: w428 -> [_ w436]
          tunnel: w431 -> [_ w435]
          tunnel: [w433 w434] -> w429
          frame False {
          }
          frame True {
            n232 = property class="Ring (strict)"(reference=w436, "Strings []"=w435) -> ()  [unwired: 1 in, 2 out]
          }
        }
        n233 = local write "folder --OK"(w429) -> ()
      }
      event "sweep folder 1": Mouse Enter {
        n234 = event-data() -> ()  [unwired: 1 in, 1 out]
        n235 = call "list - get folder names.vi"("Numeric sort?"=TRUE, "folder path"=w440) -> ("Array"=w441:string[], "OK"=w442:bool)  [unwired: 8 in]
        n236 = case shown="True" w442 {
          selector: w442 -> [w443 w444]
          tunnel: w438 -> [_ w446]
          tunnel: w441 -> [_ w445]
          tunnel: [w443 w444] -> w439
          frame False {
          }
          frame True {
            n237 = property class="Ring (strict)"(reference=w446, "Strings []"=w445) -> ()  [unwired: 1 in, 2 out]
          }
        }
        n238 = local write "folder --OK"(w439) -> ()
      }
      event "sweep folder 1": Value Change {
        n239 = event-data() -> ()  [unwired: 1 in, 6 out]
        n240 = local read "sweep folder 1"() -> (w452:u16)
        n241 = property class="Ring (strict)"(reference=w454) -> ("Strings []"=w453:string[])  [unwired: 1 in, 2 out]
        n242 = Index Array(array=w453, index=w452) -> (element=w450:string)
        n243 = Generate User Event(user event=w447, event data cluster="update file path 1" ("event data")) -> ()  [unwired: 1 in, 2 out]
        n244 = Build Path(base path=w451, name or relative path=w450) -> (appended path=w449:path)
        n245 = local write "folder 1"(w449) -> ()
      }
      event Value Change {
        n246 = event-data() -> ()  [unwired: 1 in, 1 out]
        n247 = Generate User Event(user event=w455, event data cluster="update fit" ("event data")) -> ()  [unwired: 1 in, 2 out]
      }
      event "sweep folder 2": Value Change {
        n248 = event-data() -> ()  [unwired: 1 in, 6 out]
        n249 = property class="Ring (strict)"(reference=w459) -> ("Strings []"=w464:string[])  [unwired: 1 in, 2 out]
        n250 = local read "sweep folder 2"() -> (w463:u16)
        n251 = Index Array(array=w464, index=w463) -> (element=w461:string)
        n252 = Build Path(base path=w462, name or relative path=w461) -> (appended path=w460:path)
        n253 = Generate User Event(user event=w457, event data cluster="update file path 2" ("event data")) -> ()  [unwired: 1 in, 2 out]
        n254 = local write "folder 2"(w460) -> ()
      }
      event "Plot: field vs time": Cursor Move {
        n255 = event-data() -> ()  [unwired: 1 in, 5 out]
        n256 = call "replace cursor - plot ref - V1.vi"("action"=enum16{"", "read", "write"}."read", "Plot ref in"=w472) -> ("read X"=w471:dbl)  [unwired: 7 in, 2 out]
        n257 = call "kim-read file -one.vi"("Numeric Control"=0, "container action"=container_action."get") -> ("time array"=w467:dbl[])  [unwired: 10 in, 7 out]
        n258 = Threshold 1D Array(2:w471, 3:w467) -> (0:w469:dbl)  [unwired: 1 in]
        n259 = local write "current index"(w469) -> ()
        n260 = local write "time (min)"(w471) -> ()
        n261 = Generate User Event(user event=w470, event data cluster="update cursor -- from field plot " ("event data")) -> ()  [unwired: 1 in, 2 out]
      }
      event "Plot: temp vs time": Cursor Move {
        n262 = event-data() -> ("CursIdx"=w477:i32)  [unwired: 1 in, 4 out]
        n263 = case shown="1..3, Default" w477 {
          selector: w477 -> [w481 _]
          tunnel: w478 -> [_ w504]
          tunnel: w476 -> [_ w499]
          tunnel: w475 -> [w479 _]
          tunnel: w474 -> [w480 _]
          frame 1..3, Default {
            n264 = call "cursor window logic V2.vi"("CursIdx"=w481, "cursor window action"=cursor_window_action."cursor moves", "cursor window in"=w479) -> ("cursor window out"=w496:T8)  [unwired: 7 in, 1 out]
            n265 = Unbundle By Name(w496) -> ("left"=w493:dbl, "right"=w491:dbl)
            n266 = call "kim-read file -one.vi"("Numeric Control"=0, "container action"=container_action."get") -> ("Temperature (K) Array"=w488:dbl[], "time array"=w492:dbl[])  [unwired: 10 in, 6 out]
            n267 = Threshold 1D Array(2:w491, 3:w492) -> (0:w489:dbl)  [unwired: 1 in]
            n268 = Threshold 1D Array(2:w493, 3:w492) -> (0:w490:dbl)  [unwired: 1 in]
            n269 = Index Array(array=w488, index #1=w490, index #2=w489) -> (element #1=w487:dbl, element #2=w486:dbl)
            n270 = call "Q -- range multiplier -- real.vi"("factor"=1.0, "lower"=w487, "upper"=w486) -> ("center"=w482:dbl, "window"=w484:dbl)  [unwired: 5 in, 2 out]
            n271 = Absolute Value(x=w484) -> (abs(x)=w483:dbl)
            n272 = call "cursor window logic V2.vi"("cursor window action"=cursor_window_action."change cen&win", "window"=w483, "center"=w482, "cursor window in"=w480) -> ()  [unwired: 6 in, 2 out]
          }
          frame 0 {
            n273 = call "replace cursor - plot ref - V1.vi"("action"=enum16{"", "read", "write"}."read", "Plot ref in"=w504) -> ("read X"=w506:dbl)  [unwired: 7 in, 2 out]
            n274 = call "kim-read file -one.vi"("Numeric Control"=0, "container action"=container_action."get") -> ("time array"=w502:dbl[])  [unwired: 10 in, 7 out]
            n275 = Threshold 1D Array(2:w506, 3:w502) -> (0:w505:dbl)  [unwired: 1 in]
            n276 = local write "current index"(w505) -> ()
            n277 = local write "time (min)"(w506) -> ()
            n278 = Generate User Event(user event=w499, event data cluster="update cursor -- from temperature plot" ("event data")) -> ()  [unwired: 1 in, 2 out]
          }
        }
      }
      event "plot (p)": Value Change {
        n279 = event-data() -> ()  [unwired: 1 in, 2 out]
        n280 = Generate User Event(user event=w510, event data cluster="plot" ("event data")) -> ()  [unwired: 1 in, 2 out]
      }
      event "open (o)": Value Change {
        n281 = event-data() -> ()  [unwired: 1 in, 2 out]
        n282 = Generate User Event(user event=w513, event data cluster="read file" ("event data")) -> ()  [unwired: 1 in, 2 out]
      }
    }
    n283 = Wait (ms)(milliseconds to wait=u32 1) -> ()  [unwired: 1 out]
  }
  n284 = control-ref of="timer  \"update\""() -> (w30:refnum<vi>)
  n285 = call "slider timer .vi"("action"=countdown_control."start", "timer ref"=w30) -> ("timer out"=w29:refnum<vi>)  [unwired: 7 in, 2 out]
  n286 = while {
    shift-right: [w518] -> _
    shift-left: w29 -> [w519]
    tunnel: w28 -> [w515]
    stop <- FALSE stop-if-true
    n287 = case shown="\"timer ON\", Default" "Tab: timer" {
      tunnel: w519 -> [w523 w527]
      tunnel: [w522 w527] -> w518
      tunnel: w515 -> [w520 _]
      frame "timer ON", Default {
        n288 = call "slider timer .vi"("action"=countdown_control."check", "timer ref"=w523) -> ("tic"=w521:bool, "timer out"=w522:refnum<vi>)  [unwired: 7 in, 1 out]
        n289 = case shown="True" w521 {
          tunnel: w520 -> [_ w525]
          frame False {
          }
          frame True {
            n290 = Generate User Event(user event=w525, event data cluster="read file" ("event data")) -> ()  [unwired: 1 in, 2 out]
          }
        }
      }
      frame "timer OFF" {
      }
    }
    n291 = Wait (ms)(milliseconds to wait=u32 123) -> ()  [unwired: 1 out]
  }
